vi "test_lvpid_get_advanced_error.vi"   [LabVIEW 2014]
uses:
  <vilib>/addons/control/pid/NI_PID_pid.lvlib
types:
  T1 = enum16{"open", "replace", "create", "open or create", "replace or create", "replace or create with confirmation"}
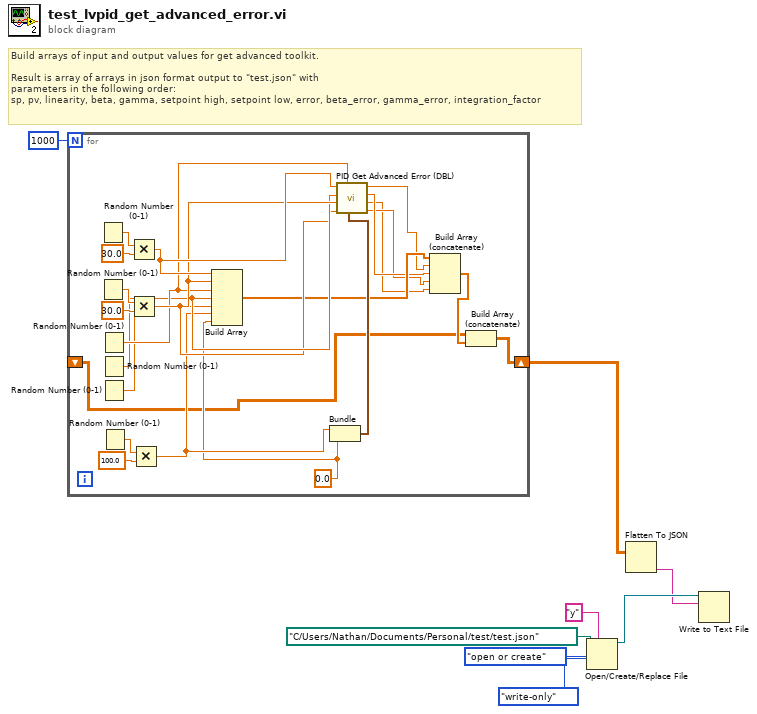
[diagram p0: block diagram]
diagram:
  # "Build arrays of input and output values for get advanced toolkit. \n\nResult is array of arrays in json format output to \"test.json\" with\nparameters in the following order:\nsp, pv, linearity, beta, gamma, setpoint high, setpoint low, error, beta_error, gamma_error, integration_factor"
  n1 = for {
    N: 1000 -> [_]
    shift-right: [w11] -> w1
    shift-left: _ -> [w9]
    w17 = 0.0
    n2 = Random Number (0-1)() -> (number: 0 to 1=w30:dbl)
    n3 = Random Number (0-1)() -> (number: 0 to 1=w28:dbl)
    n4 = Random Number (0-1)() -> (number: 0 to 1=w22:dbl)
    n5 = Random Number (0-1)() -> (number: 0 to 1=w21:dbl)
    n6 = Random Number (0-1)() -> (number: 0 to 1=w20:dbl)
    n7 = Random Number (0-1)() -> (number: 0 to 1=w26:dbl)
    n8 = Multiply(x=w30, y=30.0) -> (x*y=w24:dbl)
    n9 = Multiply(x=w28, y=30.0) -> (x*y=w23:dbl)
    n10 = Multiply(x=w26, y=100.0) -> (x*y=w19:dbl)
    n11 = Build Array(w24, w23, w22, w21, w20, w19, w17) -> (w16:dbl[])
    n12 = Bundle(w19, w17) -> (w18:cluster{dbl, dbl})  [unwired: 1 in]
    n13 = call <vilib>:"PID Get Advanced Error (DBL).vi"("setpoint range"=w18, "linearity"=w22, "Gamma"=w20, "process variable"=w23, "beta"=w21, "setpoint"=w24) -> ("error with gamma"=w13:dbl, "non-linear integral action"=w12:dbl, "error with beta"=w14:dbl, "error"=w15:dbl)  [unwired: 2 out]
    n14 = Build Array (concatenate)(w16, w15, w14, w13, w12) -> (w10:dbl[])
    n15 = Build Array (concatenate)(w9, w10) -> (w11:dbl[][])
  }
  n16 = Open/Create/Replace File(file path (use dialog)=path "C:/Users/Nathan/Documents/Personal/test/test.json", prompt="y", operation (0:open)=T1."open or create", access (0:read/write)=enum16{"read/write", "read-only", "write-only"}."write-only") -> (refnum out=w7:refnum<file>)  [unwired: 2 in, 2 out]
  n17 = Flatten To JSON(anything=w1) -> (JSON string=w6:string)  [unwired: 2 in, 1 out]
  n18 = Write to Text File(file (use dialog)=w7, text=w6) -> ()  [unwired: 2 in, 3 out]
